vi "Post-Install Action.vi"(10 "Variant":variant) -> (0 "error out":errorcluster)   [LabVIEW 2014]
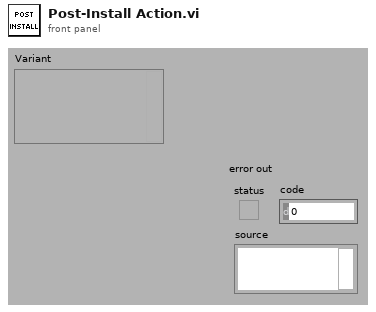
[diagram p1: front panel]
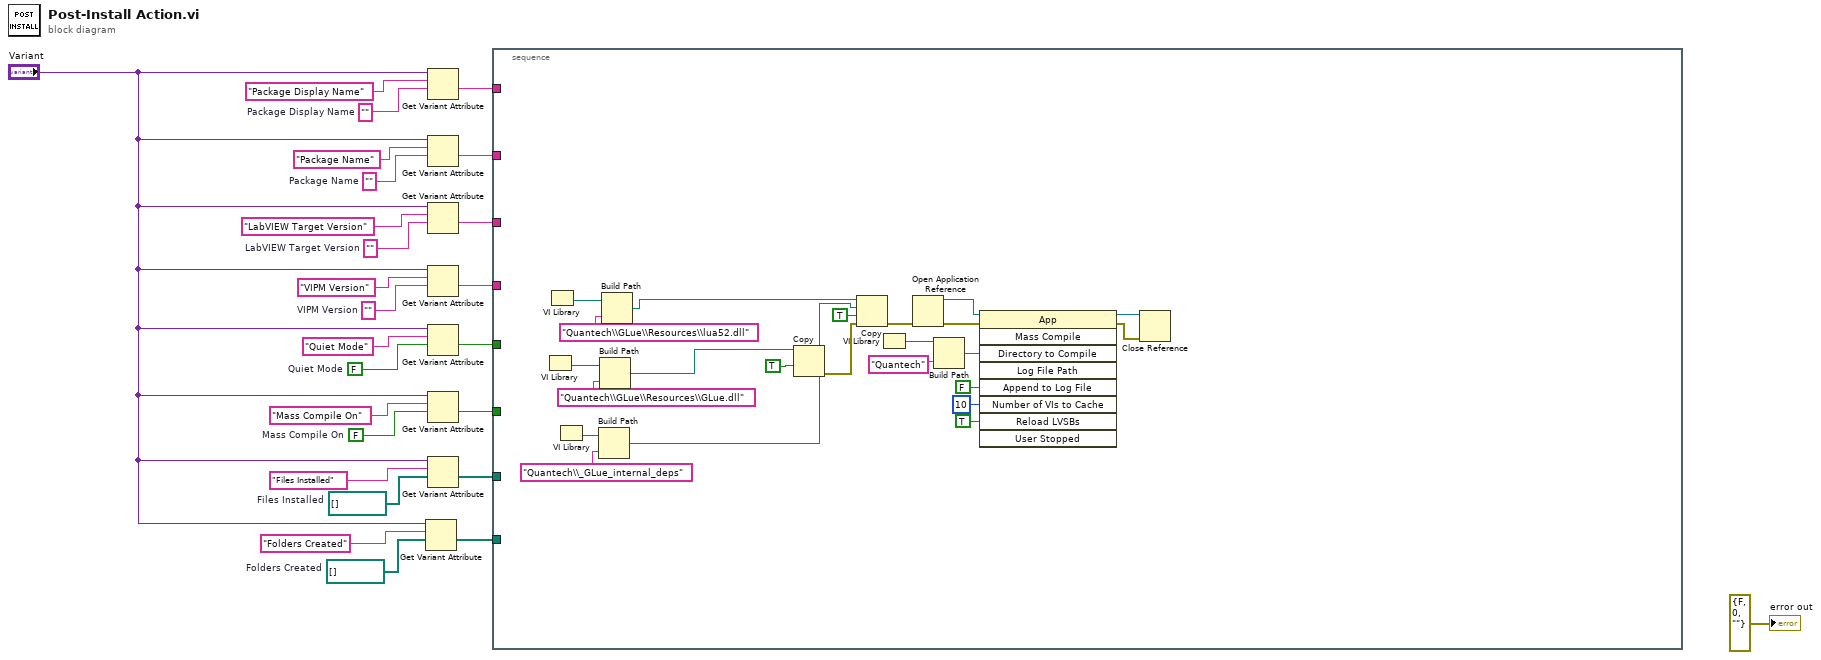
[diagram p0: block diagram]
diagram:
  w1 = path[] []  # Folders Created
  w2 = path[] []  # Files Installed
  w8 = FALSE  # Mass Compile On
  w9 = ""  # Package Display Name
  w16 = FALSE  # Quiet Mode
  w19 = ""  # VIPM Version
  w21 = ""  # LabVIEW Target Version
  w23 = ""  # Package Name
  n1 = Get Variant Attribute(Variant="Variant", name="Folders Created", default value (empty Variant)=w1) -> (value=w6:path[])  [unwired: 1 in, 3 out]
  n2 = Get Variant Attribute(Variant="Variant", name="Package Display Name", default value (empty Variant)=w9) -> (value=w15:string)  [unwired: 1 in, 3 out]
  n3 = Get Variant Attribute(Variant="Variant", name="Package Name", default value (empty Variant)=w23) -> (value=w14:string)  [unwired: 1 in, 3 out]
  n4 = Get Variant Attribute(Variant="Variant", name="LabVIEW Target Version", default value (empty Variant)=w21) -> (value=w13:string)  [unwired: 1 in, 3 out]
  n5 = Get Variant Attribute(Variant="Variant", name="VIPM Version", default value (empty Variant)=w19) -> (value=w12:string)  [unwired: 1 in, 3 out]
  n6 = Get Variant Attribute(Variant="Variant", name="Quiet Mode", default value (empty Variant)=w16) -> (value=w11:bool)  [unwired: 1 in, 3 out]
  n7 = Get Variant Attribute(Variant="Variant", name="Mass Compile On", default value (empty Variant)=w8) -> (value=w10:bool)  [unwired: 1 in, 3 out]
  n8 = Get Variant Attribute(Variant="Variant", name="Files Installed", default value (empty Variant)=w2) -> (value=w5:path[])  [unwired: 1 in, 3 out]
  n9 = stacked-sequence {
    tunnel: w15 -> [_]
    tunnel: w14 -> [_]
    tunnel: w13 -> [_]
    tunnel: w12 -> [_]
    tunnel: w11 -> [_]
    tunnel: w10 -> [_]
    tunnel: w5 -> [_]
    tunnel: w6 -> [_]
    frame #0 {
      n10 = VI Library() -> (path=w37:path)
      n11 = VI Library() -> (path=w38:path)
      n12 = VI Library() -> (path=w33:path)
      n13 = Build Path(base path=w33, name or relative path="Quantech\\_GLue_internal_deps") -> (appended path=w29:path)
      n14 = Build Path(base path=w37, name or relative path="Quantech\\GLue\\Resources\\GLue.dll") -> (appended path=w30:path)
      n15 = Build Path(base path=w38, name or relative path="Quantech\\GLue\\Resources\\lua52.dll") -> (appended path=w31:path)
      n16 = Copy(9:TRUE ("overwrite (F)"), 10:w29, 11:w30) -> (0:w28:errorcluster)  [unwired: 2 in, 2 out]
      n17 = Copy(8:w28, 9:TRUE ("overwrite (F)"), 10:w29, 11:w31) -> (0:w27:errorcluster)  [unwired: 1 in, 2 out]
      n18 = VI Library() -> (path=w42:path)
      n19 = Open Application Reference(8:w27) -> (0:w48:errorcluster, 3:w49:refnum<vi>)  [unwired: 3 in]
      n20 = Build Path(base path=w42, name or relative path="Quantech") -> (appended path=w40:path)
      n21 = invoke class="App" method="Mass Compile"(reference=w49, error in=w48, "Directory to Compile"=w40, "Append to Log File"=FALSE, "Number of VIs to Cache"=u32 10, "Reload LVSBs"=TRUE) -> (reference out=w44:refnum<vi>, error out=w43:errorcluster)  [unwired: 3 in, 7 out]
      n22 = Close Reference(reference=w44, error in (no error)=w43) -> ()  [unwired: 1 out]
    }
  }
  "error out" <- errorcluster {"status"=FALSE, "code"=0, "source"=""} ("error out")
